vi "Ripple-carry adder.vi"(2 "B":bool[](array[boolean]), 3 "A":bool[](array[boolean]), 4 "c in":bool) -> (0 "c out":bool, 1 "S":bool[](array[boolean]))   [LabVIEW 2012]
panel:
  out "s3":bool
  out "s2":bool
  out "s1":bool
  out "s0":bool
  in  "B3":bool
  in  "A3":bool
  in  "B2":bool
  in  "A2":bool
  in  "B1":bool
  in  "A1":bool
  in  "B0":bool
  in  "A0":bool
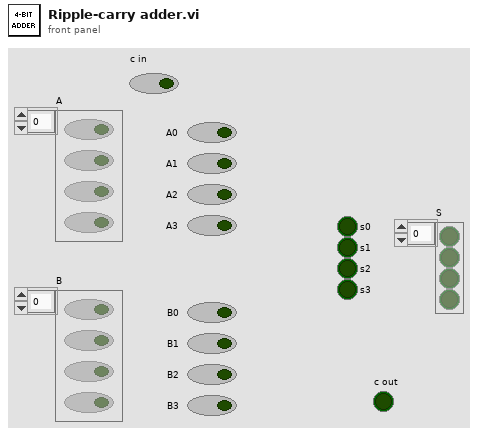
[diagram p1: front panel]
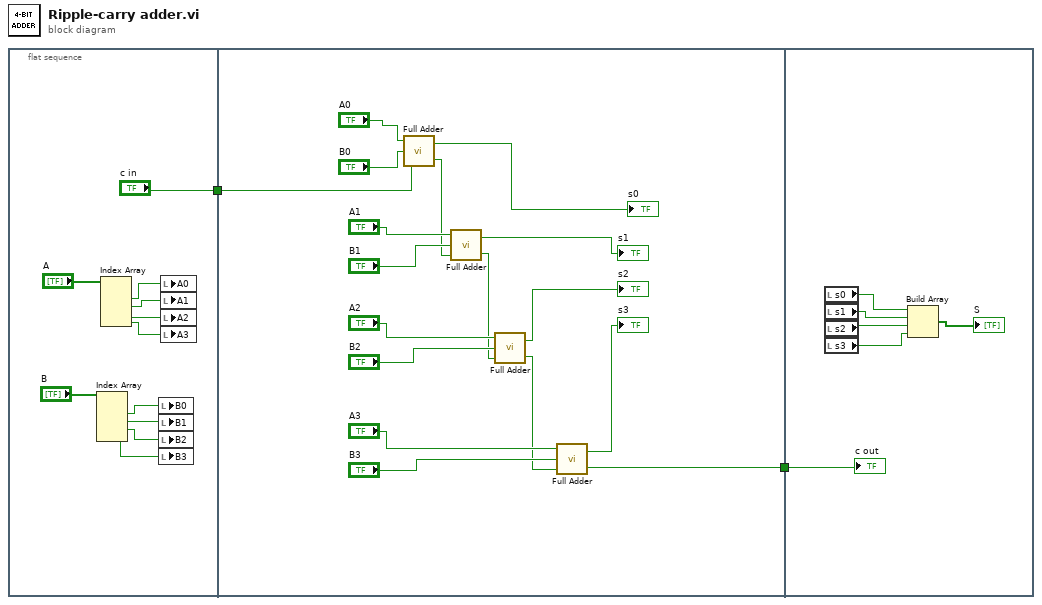
[diagram p0: block diagram]
diagram:
  n1 = flat-sequence {
    tunnel: ["c in"] -> w1
    tunnel: [w15] -> w2
    tunnel: w1 -> [w14]
    tunnel: w2 -> [w31]
    frame #0 {
      n2 = Index Array(array="B") -> (element #1=w7:bool, element #2=w6:bool, element #3=w5:bool, element #4=w4:bool)  [unwired: 4 in]
      n3 = Index Array(array="A") -> (element #1=w11:bool, element #2=w10:bool, element #3=w9:bool, element #4=w8:bool)  [unwired: 4 in]
      n4 = local write "B0"(w7) -> ()
      n5 = local write "B1"(w6) -> ()
      n6 = local write "B2"(w5) -> ()
      n7 = local write "B3"(w4) -> ()
      n8 = local write "A0"(w11) -> ()
      n9 = local write "A1"(w10) -> ()
      n10 = local write "A2"(w9) -> ()
      n11 = local write "A3"(w8) -> ()
    }
    frame #1 {
      n12 = call "Full Adder.vi"("c in"=w14, "b"="B0", "a"="A0") -> ("c out"=w18:bool, "s"=→"s0":bool)
      n13 = call "Full Adder.vi"("c in"=w18, "b"="B1", "a"="A1") -> ("c out"=w17:bool, "s"=→"s1":bool)
      n14 = call "Full Adder.vi"("c in"=w17, "b"="B2", "a"="A2") -> ("c out"=w16:bool, "s"=→"s2":bool)
      n15 = call "Full Adder.vi"("c in"=w16, "b"="B3", "a"="A3") -> ("c out"=w15:bool, "s"=→"s3":bool)
    }
    frame #2 {
      n16 = local read "s0"() -> (w36:bool)
      n17 = local read "s1"() -> (w35:bool)
      n18 = local read "s2"() -> (w34:bool)
      n19 = local read "s3"() -> (w33:bool)
      n20 = Build Array(w36, w35, w34, w33) -> (→"S":bool[])
      "c out" <- w31
    }
  }
